vi "SmartSEM Remote API set SEM parameters.vi"(6 "Det Info":T1={"Brightness A"=40.0, "Contrast A"=26.0, "Detector B name"="ESB @ 1.0 kV", "Brightness B"=40.0, "Contrast B"=40.0, "Detector C name"="PMT @ 6.0", "Detector D name"="Detector D"}, 8 "error in":errorcluster, 9 "Scan Para":T2={"X resolution"=4096, "Y resolution"=2048, "X center (um)"=0.0, "Y center (um)"=0.0, "X size (V)"=20.0, "X size auto"=TRUE, "X stig"=0.0, "Y stig"=0.0, "X aln"=0.0, "Y aln"=0.0, "Scan rate (Hz)"=10000000, "Oversampling"=10, "Oversampling auto"=TRUE, "Frame line rampdown ratio"=0.1, "Pixel size (nm)"=5.0, "WD"=4.0} {"WD" format="%#_7g"; "Frame line rampdown ratio" min=-1 max=1 step=0.05 format="%.2g"; "Scan rate (Hz)" max=4000000 format="%.2e"}, 10 "SEM Options":T3={"GetInfo"=TRUE, "Set Det A para"=TRUE, "Set WD"=FALSE, "Set Mag"=TRUE, "Set stig"=FALSE, "Set aln"=FALSE, "Display"=TRUE, "Save"=TRUE, "8-bit"=TRUE, "Detector A"=TRUE, "Detector B"=FALSE, "Detector C"=FALSE, "Detector D"=FALSE, "Inverse A"=FALSE, "Inverse B"=FALSE, "Inverse C"=FALSE, "Inverse D"=FALSE, "Inverse PNG"=TRUE, "Freeze"=TRUE, "PNG only"=FALSE, "Upload"=FALSE, "Delete after upload"=FALSE}, 11 "ActiveX Container":refnum<k7>(container)) -> (0 "error out":errorcluster, 3 "reference out":refnum<k7>)   [LabVIEW 2018]
panel:
  out "Det A Type":string="InLens"
  out "Grid voltage":sgl
  out "Det B Type":string
  out "Set Mag":bool
  out "Set WD":bool
  out "Set aln":bool
  out "Set stig":bool
  out "Set Det para":bool
  out "Mag":sgl=285.0
  out "WD":sgl=0.0036
  out "Y aln":sgl=2.5
  out "X aln":sgl=1.5
  out "Y stig":sgl=1.0
  out "X stig":sgl=1.0
  out "Det A Contrast":sgl=45.0
  out "Det A Brightness":sgl=35.0
  out "Det B Contrast":sgl=40.0
  out "Det B Brightness":sgl=30.0
  # "Detector A"
  # "Det"
  # "after"
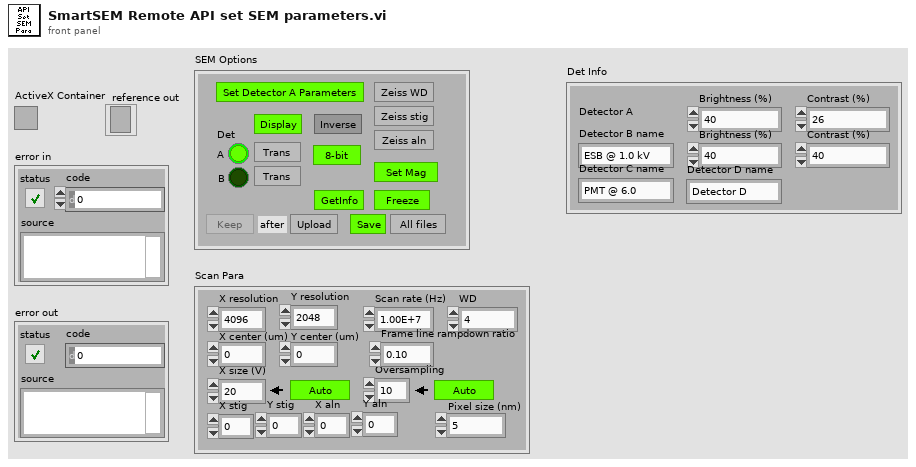
[diagram p1: front panel]
types:
  T1 = cluster{"Brightness A":dbl, "Contrast A":dbl, "Detector B name":string, "Brightness B":dbl, "Contrast B":dbl, "Detector C name":string, "Detector D name":string}
  T2 = cluster{"X resolution":u32, "Y resolution":u32, "X center (um)":sgl, "Y center (um)":sgl, "X size (V)":dbl, "X size auto":bool, "X stig":sgl, "Y stig":sgl, "X aln":sgl, "Y aln":sgl, "Scan rate (Hz)":u32, "Oversampling":u32, "Oversampling auto":bool, "Frame line rampdown ratio":sgl, "Pixel size (nm)":sgl, "WD":sgl}
  T3 = cluster{"GetInfo":bool, "Set Det A para":bool, "Set WD":bool, "Set Mag":bool, "Set stig":bool, "Set aln":bool, "Display":bool, "Save":bool, "8-bit":bool, "Detector A":bool, "Detector B":bool, "Detector C":bool, "Detector D":bool, "Inverse A":bool, "Inverse B":bool, "Inverse C":bool, "Inverse D":bool, "Inverse PNG":bool, "Freeze":bool, "PNG only":bool, "Upload":bool, "Delete after upload":bool}
  T4 = enum16{"SEM", "FIB", "Mill", "SEM + FIB", "Mill + SEM", "Drift SEM", "Drift FIB", "None", "Ext", "Ext + SEM"}
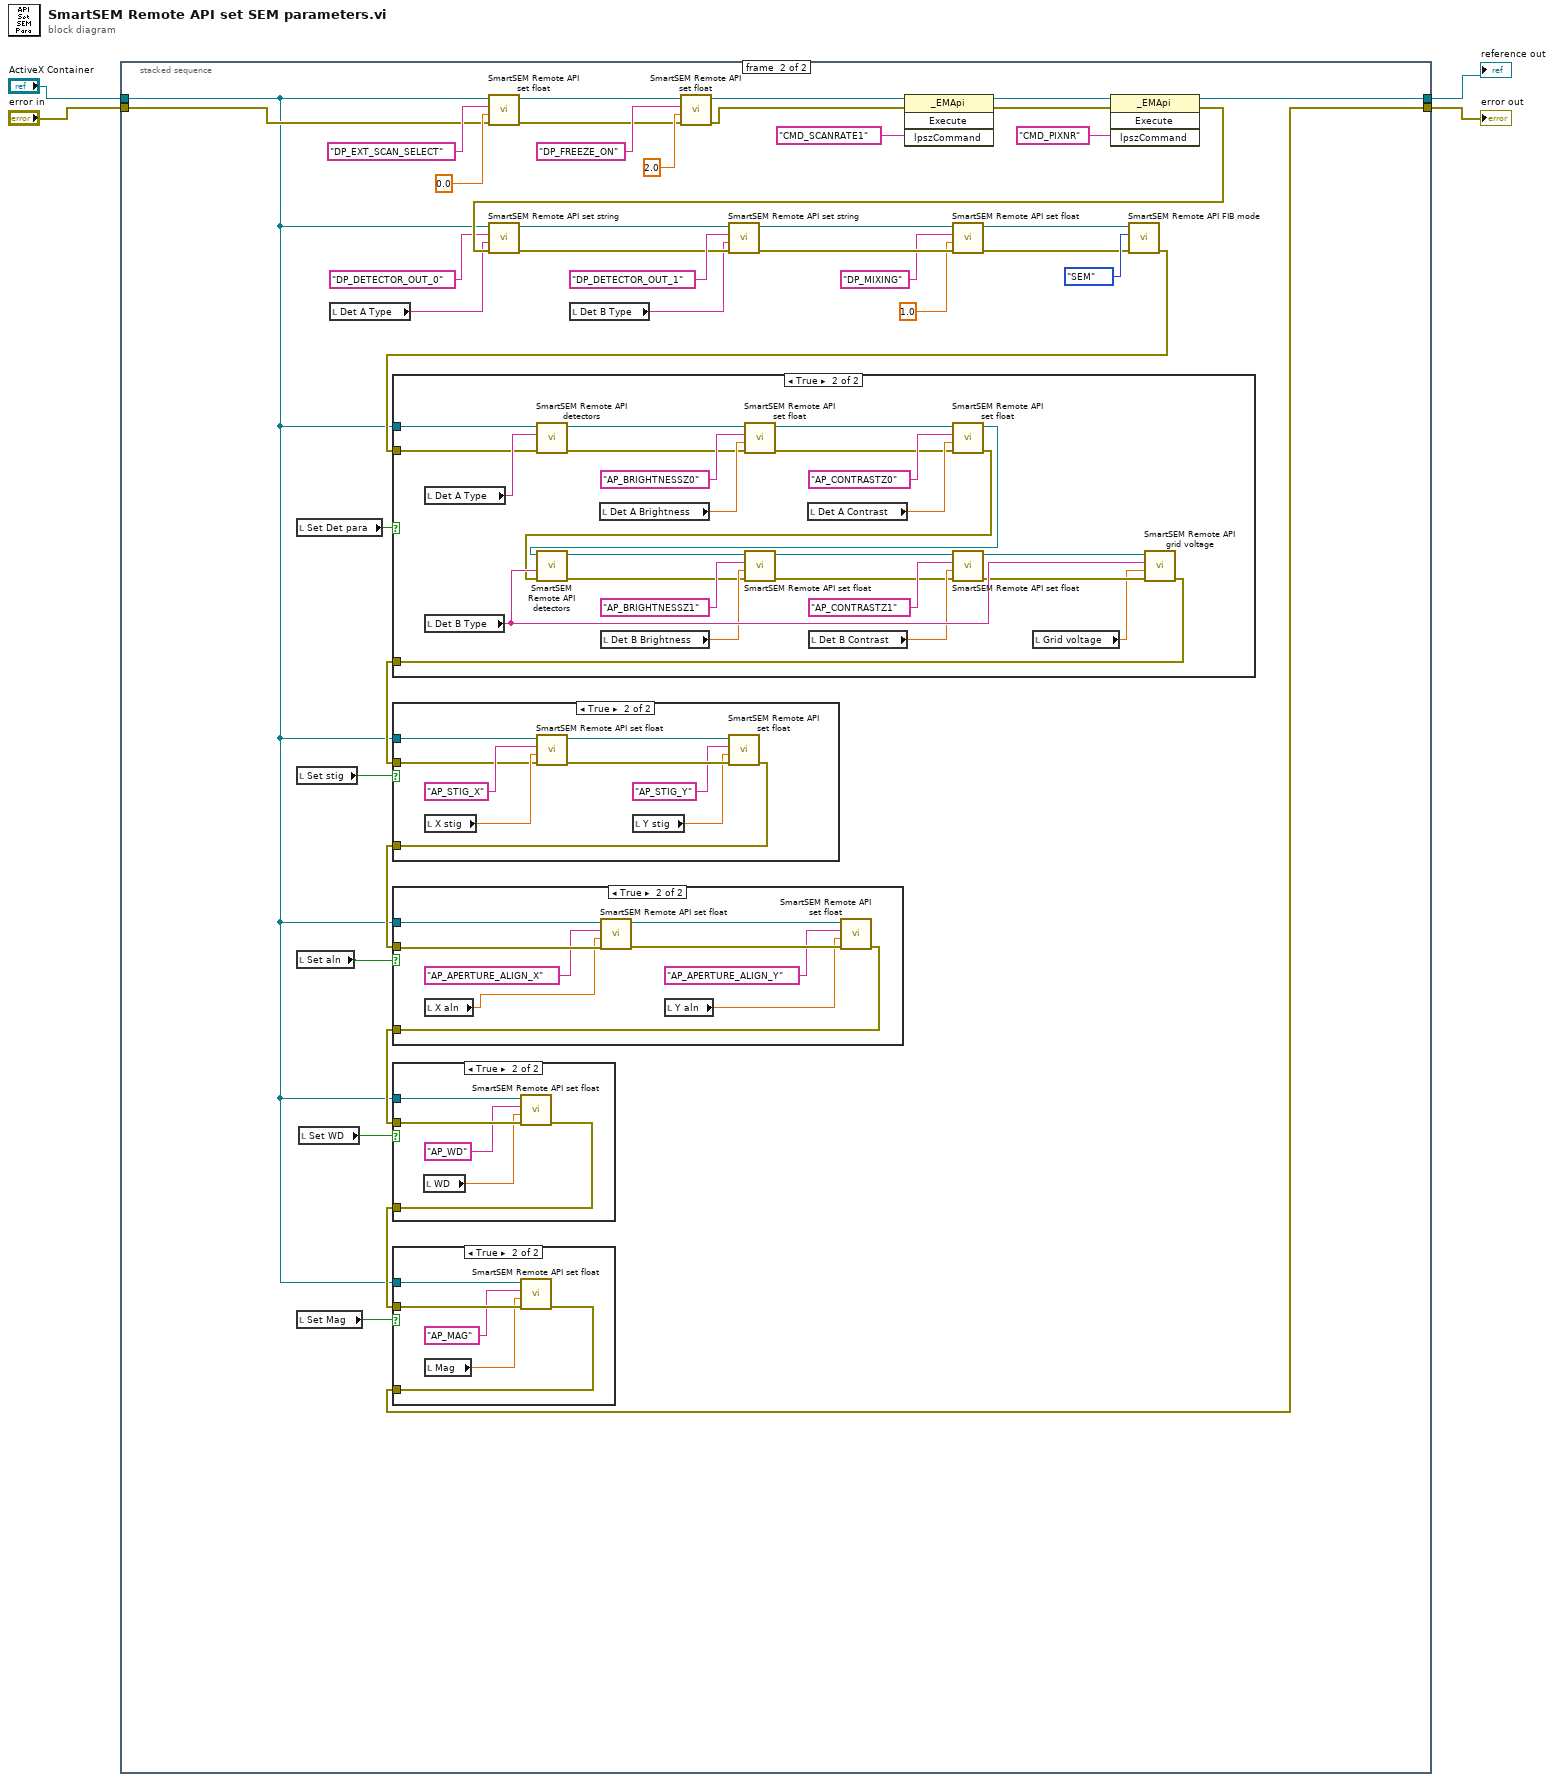
[diagram p0: block diagram]
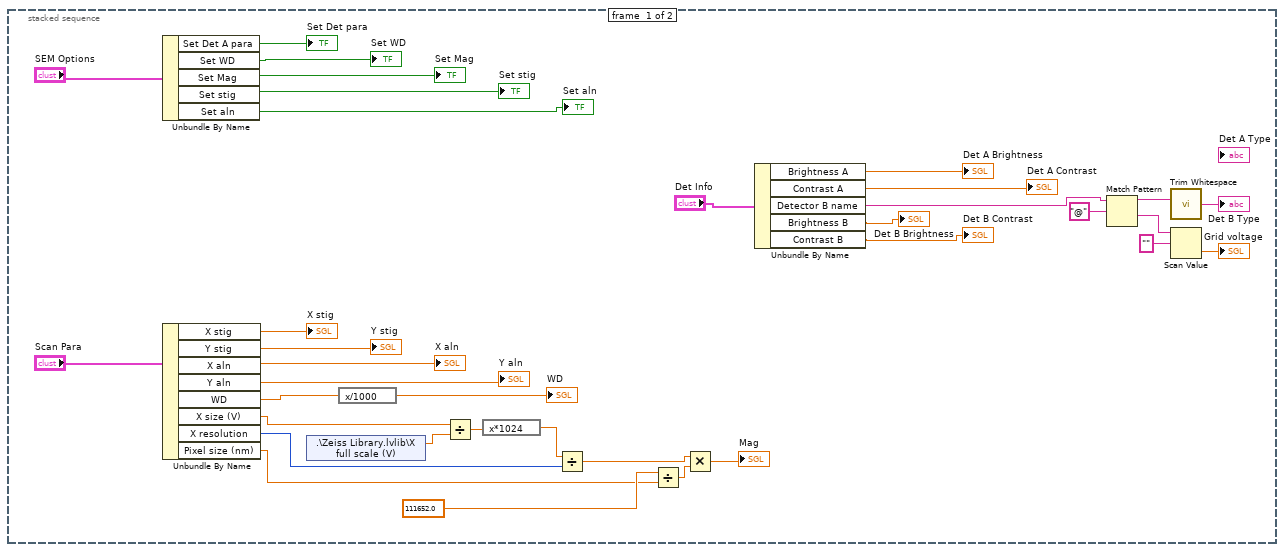
[diagram p2: hidden frame]
diagram:
  n1 = stacked-sequence {
    tunnel: [_ w72] -> w4
    tunnel: [_ w56] -> w2
    tunnel: "error in" -> [_ w41]
    tunnel: "ActiveX Container" -> [_ w40]
    frame #0 {
      n2 = Unbundle By Name("SEM Options") -> ("Set Det A para"=→"Set Det para":bool, "Set WD"=→"Set WD":bool, "Set Mag"=→"Set Mag":bool, "Set stig"=→"Set stig":bool, "Set aln"=→"Set aln":bool)
      n3 = Unbundle By Name("Scan Para") -> ("X stig"=→"X stig":sgl, "Y stig"=→"Y stig":sgl, "X aln"=→"X aln":sgl, "Y aln"=→"Y aln":sgl, "WD"=w28:sgl, "X size (V)"=w25:dbl, "X resolution"=w24:u32, "Pixel size (nm)"=w20:sgl)
      n4 = shared-variable ".\\Zeiss Library.lvlib\\X full scale (V)"() -> (w13:sgl)  [unwired: 1 in, 1 out]
      n5 = expression code="x/1000"(w28) -> (→"WD":sgl)
      n6 = Divide(x=w25, y=w13) -> (x/y=w26:dbl)
      n7 = expression code="x*1024"(w26) -> (w27:dbl)
      n8 = Divide(x=w27, y=w24) -> (x/y=w21:dbl)
      n9 = Divide(x=111652.0, y=w20) -> (x/y=w23:dbl)
      n10 = Multiply(x=w21, y=w23) -> (x*y=→"Mag":dbl)
      n11 = Unbundle By Name("Det Info") -> ("Brightness A"=→"Det A Brightness":dbl, "Contrast A"=→"Det A Contrast":dbl, "Detector B name"=w10:string, "Brightness B"=→"Det B Brightness":dbl, "Contrast B"=→"Det B Contrast":dbl)
      n12 = Match Pattern(string=w10, regular expression="@") -> (before substring=w9:string, after substring=w6:string)  [unwired: 1 in, 2 out]
      n13 = call <vilib>:"Trim Whitespace.vi"("string"=w9) -> ("trimmed string"=→"Det B Type":string)  [unwired: 1 in]
      n14 = Scan Value(string=w6, format string="") -> (value=→"Grid voltage":dbl)  [unwired: 1 in, 1 out]
    }
    frame #1 {
      n15 = local read "Set Det para"() -> (w78:bool)
      n16 = local read "Set stig"() -> (w77:bool)
      n17 = local read "Set aln"() -> (w76:bool)
      n18 = local read "Set Mag"() -> (w74:bool)
      n19 = local read "Set WD"() -> (w75:bool)
      n20 = local read "Det A Type"() -> (w65:string)
      n21 = call "SmartSEM Remote API set float.vi"("error in"=w41, "vValue"=sgl 0.0 ("Freeze on"), "lpszParam"="DP_EXT_SCAN_SELECT" ("lpszCommand"), "ActiveX Container"=w40) -> ("error out"=w48:errorcluster, "reference out"=w49:refnum<k7>)  [unwired: 6 in]
      n22 = local read "Det B Type"() -> (w61:string)
      n23 = call "SmartSEM Remote API set float.vi"("error in"=w48, "vValue"=sgl 2.0 ("Freeze on"), "lpszParam"="DP_FREEZE_ON" ("lpszCommand"), "ActiveX Container"=w49) -> ("error out"=w58:errorcluster, "reference out"=w59:refnum<k7>)  [unwired: 6 in]
      n24 = invoke class="_EMApi" method="Execute"(reference=w59, error in=w58, "lpszCommand"="CMD_SCANRATE1") -> (reference out=w53:refnum<k7>, error out=w52:errorcluster)  [unwired: 1 in, 2 out]
      n25 = invoke class="_EMApi" method="Execute"(reference=w53, error in=w52, "lpszCommand"="CMD_PIXNR") -> (reference out=w72:refnum<k7>, error out=w67:errorcluster)  [unwired: 1 in, 2 out]
      n26 = call "SmartSEM Remote API set string.vi"("error in"=w67, "vValue"=w65, "lpszParam"="DP_DETECTOR_OUT_0" ("lpszCommand"), "ActiveX Container"=w40) -> ("error out"=w62:errorcluster, "reference out"=w63:refnum<k7>)  [unwired: 6 in]
      n27 = call "SmartSEM Remote API set string.vi"("error in"=w62, "vValue"=w61, "lpszParam"="DP_DETECTOR_OUT_1" ("lpszCommand"), "ActiveX Container"=w63) -> ("error out"=w46:errorcluster, "reference out"=w47:refnum<k7>)  [unwired: 6 in]
      n28 = call "SmartSEM Remote API set float.vi"("error in"=w46, "vValue"=sgl 1.0 ("Freeze on"), "lpszParam"="DP_MIXING" ("lpszCommand"), "ActiveX Container"=w47) -> ("error out"=w43:errorcluster, "reference out"=w42:refnum<k7>)  [unwired: 6 in]
      n29 = call "SmartSEM Remote API FIB mode.vi"("error in"=w43, "FIB mode"=T4."SEM", "ActiveX Container"=w42) -> ("error out"=w50:errorcluster)  [unwired: 7 in, 1 out]
      n30 = case shown="True" w78 {
        tunnel: w40 -> [_ w129]
        tunnel: w50 -> [w112 w128]
        tunnel: [w112 w113] -> w71
        frame False {
        }
        frame True {
          n31 = local read "Det A Type"() -> (w138:string)
          n32 = local read "Det B Type"() -> (w127:string)
          n33 = call "SmartSEM Remote API detectors.vi"("error in"=w128, "Det A Type"=w138, "ActiveX Container"=w129) -> ("error out"=w130:errorcluster, "reference out"=w131:refnum<k7>)  [unwired: 7 in]
          n34 = local read "Det A Brightness"() -> (w136:sgl)
          n35 = local read "Det B Brightness"() -> (w126:sgl)
          n36 = call "SmartSEM Remote API set float.vi"("error in"=w130, "vValue"=w136, "lpszParam"="AP_BRIGHTNESSZ0" ("lpszCommand"), "ActiveX Container"=w131) -> ("error out"=w132:errorcluster, "reference out"=w137:refnum<k7>)  [unwired: 6 in]
          n37 = local read "Det A Contrast"() -> (w134:sgl)
          n38 = local read "Det B Contrast"() -> (w124:sgl)
          n39 = call "SmartSEM Remote API set float.vi"("error in"=w132, "vValue"=w134, "lpszParam"="AP_CONTRASTZ0" ("lpszCommand"), "ActiveX Container"=w137) -> ("error out"=w114:errorcluster, "reference out"=w115:refnum<k7>)  [unwired: 6 in]
          n40 = call "SmartSEM Remote API detectors.vi"("error in"=w114, "Det B Type"=w127, "ActiveX Container"=w115) -> ("error out"=w116:errorcluster, "reference out"=w117:refnum<k7>)  [unwired: 7 in]
          n41 = call "SmartSEM Remote API set float.vi"("error in"=w116, "vValue"=w126, "lpszParam"="AP_BRIGHTNESSZ1" ("lpszCommand"), "ActiveX Container"=w117) -> ("error out"=w120:errorcluster, "reference out"=w122:refnum<k7>)  [unwired: 6 in]
          n42 = call "SmartSEM Remote API set float.vi"("error in"=w120, "vValue"=w124, "lpszParam"="AP_CONTRASTZ1" ("lpszCommand"), "ActiveX Container"=w122) -> ("error out"=w119:errorcluster, "reference out"=w121:refnum<k7>)  [unwired: 6 in]
          n43 = local read "Grid voltage"() -> (w118:sgl)
          n44 = call "SmartSEM Remote API grid voltage.vi"("error in"=w119, "Grid voltage"=w118, "Det Type"=w127, "ActiveX Container"=w121) -> ("error out"=w113:errorcluster)  [unwired: 6 in, 1 out]
        }
      }
      n45 = case shown="True" w77 {
        tunnel: w40 -> [_ w111]
        tunnel: w71 -> [w102 w103]
        tunnel: [w102 w106] -> w70
        frame False {
        }
        frame True {
          n46 = local read "X stig"() -> (w105:sgl)
          n47 = call "SmartSEM Remote API set float.vi"("error in"=w103, "vValue"=w105, "lpszParam"="AP_STIG_X" ("lpszCommand"), "ActiveX Container"=w111) -> ("error out"=w109:errorcluster, "reference out"=w110:refnum<k7>)  [unwired: 6 in]
          n48 = local read "Y stig"() -> (w108:sgl)
          n49 = call "SmartSEM Remote API set float.vi"("error in"=w109, "vValue"=w108, "lpszParam"="AP_STIG_Y" ("lpszCommand"), "ActiveX Container"=w110) -> ("error out"=w106:errorcluster)  [unwired: 6 in, 1 out]
        }
      }
      n50 = case shown="True" w76 {
        tunnel: w40 -> [_ w101]
        tunnel: w70 -> [w92 w100]
        tunnel: [w92 w93] -> w69
        frame False {
        }
        frame True {
          n51 = local read "X aln"() -> (w99:sgl)
          n52 = call "SmartSEM Remote API set float.vi"("error in"=w100, "vValue"=w99, "lpszParam"="AP_APERTURE_ALIGN_X" ("lpszCommand"), "ActiveX Container"=w101) -> ("error out"=w96:errorcluster, "reference out"=w97:refnum<k7>)  [unwired: 6 in]
          n53 = local read "Y aln"() -> (w95:sgl)
          n54 = call "SmartSEM Remote API set float.vi"("error in"=w96, "vValue"=w95, "lpszParam"="AP_APERTURE_ALIGN_Y" ("lpszCommand"), "ActiveX Container"=w97) -> ("error out"=w93:errorcluster)  [unwired: 6 in, 1 out]
        }
      }
      n55 = case shown="True" w75 {
        tunnel: w40 -> [_ w87]
        tunnel: w69 -> [w86 w91]
        tunnel: [w86 w90] -> w68
        frame False {
        }
        frame True {
          n56 = local read "WD"() -> (w88:sgl)
          n57 = call "SmartSEM Remote API set float.vi"("error in"=w91, "vValue"=w88, "lpszParam"="AP_WD" ("lpszCommand"), "ActiveX Container"=w87) -> ("error out"=w90:errorcluster)  [unwired: 6 in, 1 out]
        }
      }
      n58 = case shown="True" w74 {
        tunnel: w40 -> [_ w85]
        tunnel: w68 -> [w80 w84]
        tunnel: [w80 w83] -> w56
        frame False {
        }
        frame True {
          n59 = local read "Mag"() -> (w82:sgl)
          n60 = call "SmartSEM Remote API set float.vi"("error in"=w84, "vValue"=w82, "lpszParam"="AP_MAG" ("lpszCommand"), "ActiveX Container"=w85) -> ("error out"=w83:errorcluster)  [unwired: 6 in, 1 out]
        }
      }
    }
  }
  "error out" <- w2
  "reference out" <- w4
